vi "Select Cleanup Objects.vi"(11 "HTTP Server.lvlib:Processing":refnum<class "Processing.lvclass">) -> (3 "Updated Inputs":refnum<class "Processing.lvclass">, 7 "Trace Message":string)   [LabVIEW 2020, in "HTTP Server.lvlib" / "Server.lvclass"]
uses:
  Server.lvclass
  Processing/Processing.lvclass
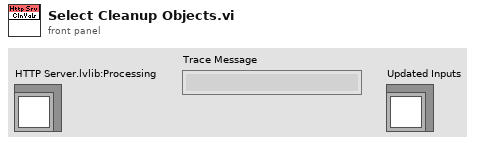
[diagram p1: front panel]
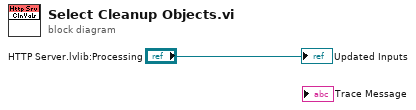
[diagram p0: block diagram]
diagram:
  "Updated Inputs" <- "HTTP Server.lvlib:Processing"
